vi "Launch as Nested.vi"(6 "Groups (Later)":refnum<class "Group.lvclass">[](array[class]), 7 "Standalone (F)":bool, 8 "error in (no error)":errorcluster, 9 "Name":string, 10 "Data Logger Config":T1={"Split Type"=enum."Count", "Split Limit"=0, "Logging Root"=path "", "Chunk Size"=1}, 11 "Parent Task in":refnum<class "Task.lvclass">) -> (0 "error out":errorcluster, 2 "API":refnum<class "DataLoggerAPI.lvclass">, 3 "Parent Task out":refnum<class "Task.lvclass">)   [LabVIEW 2020, in "VolatusDataLogger.lvlib" / "DataLogger.lvclass"]
uses:
  DataLogger.lvclass
  DataLogger.lvclass/DataLogger.ctl
  Volatus/Task/Task.lvclass
  DataLoggerAPI/DataLoggerAPI.lvclass
  lv-promises/Promises/Promise/Promise.lvclass
  C:/dev/lv20CE/relink/lv-volatus/VolatusDataLogger/DataLoggerAPI/DataLoggerAPI.lvclass
  C:/dev/lv20CE/relink/lv-volatus/Volatus/API/API.lvclass
  C:/dev/lv20CE/relink/lv-volatus/Volatus/Task/Task.lvclass
  C:/Program Files (x86)/National Instruments/LabVIEW 2020/vi.lib/ActorFramework/Actor/Actor.lvclass
  C:/dev/lv20CE/relink/lv-volatus/Volatus/APIRegistrationHandler/APIRegistrationHandler.lvclass
  C:/dev/lv20CE/relink/lv-volatus/Volatus/TaskStateHandler/TaskStateHandler.lvclass
  C:/dev/lv20CE/relink/lv-volatus/Volatus/VectoMessageHandler/VectoMessageHandler.lvclass
  C:/dev/lv20CE/relink/lv-volatus/VolatusDataLogger/DataLogger/DataLogger.lvclass
  C:/dev/lv20CE/relink/lv-volatus/Volatus/API Provider/API Provider.lvclass
  C:/dev/lv20CE/relink/lv-volatus/VolatusDataLogger/LoggingHandler/LoggingHandler.lvclass
  Split Type.ctl
  VolatusDataLogger.lvlib
  Data Logger Config.ctl
  lv-vecto/Vecto/Group/Group.lvclass
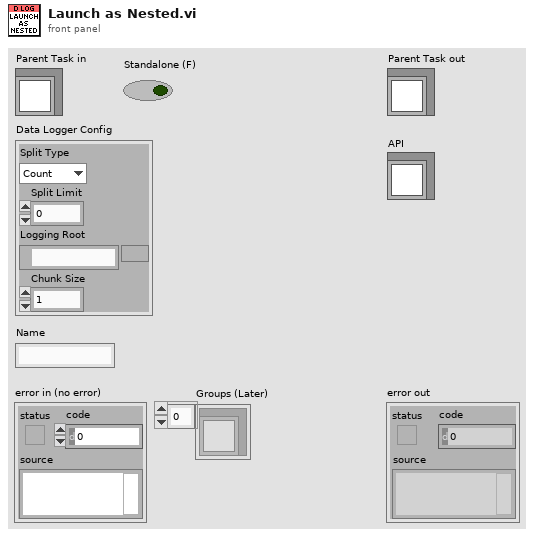
[diagram p1: front panel]
types:
  T1 = typedef "VolatusDataLogger.lvlib/Data Logger Config.ctl" = cluster{"Split Type":T2, "Split Limit":i64, "Logging Root":path, "Chunk Size":u32}
  T2 = typedef "VolatusDataLogger.lvlib/Split Type.ctl" = enum16{"Count", "Size"}
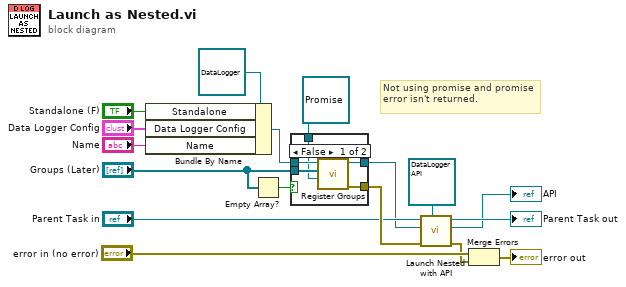
[diagram p0: block diagram]
diagram:
  # "Not using promise and promise error isn't returned."
  n1 = Bundle By Name(cluster=refnum<class "DataLogger.lvclass"> refnum ("DataLogger in"), "Standalone"="Standalone (F)", "Data Logger Config"="Data Logger Config", "Name"="Name") -> (w4:refnum<class "DataLogger.lvclass">)
  n2 = Empty Array?(array="Groups (Later)") -> (empty?=w6:bool)
  n3 = case shown="False" w6 {
    tunnel: "Groups (Later)" -> [w20 _]
    tunnel: w4 -> [w22 w23]
    tunnel: [w21 w23] -> w3
    tunnel: refnum<class "Promise.lvclass"> refnum ("Futures:Promise") -> [w19 _]
    tunnel: [w18 _] -> w17
    frame False {
      n4 = call "Register Groups.vi"("Promise"=w19, "Groups"=w20, "DataLogger in"=w22) -> ("error out"=w18:errorcluster, "DataLogger out"=w21:refnum<class "DataLogger.lvclass">)  [unwired: 7 in]
    }
    frame True {
    }
  }
  n5 = call "Launch Nested with API.vi"("API Type"=refnum<class "DataLoggerAPI.lvclass"> refnum ("API"), "error in (no error)"=w17, "Nested Task"=w3, "Task in"="Parent Task in") -> ("error out"=w9:errorcluster, "API"=→"API":refnum<class "DataLoggerAPI.lvclass">, "Task out"=→"Parent Task out":refnum<class "Task.lvclass">)  [unwired: 5 in]
  n6 = Merge Errors("error in (no error)", w9) -> (→"error out":errorcluster)
